vi "test Get Attribute as DBL2.vi"(11 "Test Case In":refnum<class "Test Config From Excel Table.lvclass">) -> (0 "error out":errorcluster, 3 "Test Case Out":refnum<class "Test Config From Excel Table.lvclass">)   [LabVIEW 2020, in "Test Config From Excel Table.lvclass"]
uses:
  Test Config From Excel Table.lvclass
  C:/Program Files/National Instruments/LabVIEW 2025/vi.lib/Astemes/LUnit/Test Case.lvclass
  Source/Config from Excel Table/Config from Excel Table.lvclass
  <vilib>/Astemes/LUnit/Test Case.lvclass/Test Case.ctl
  <vilib>/Astemes/LUnit/Test Case.lvclass
  Open-Xml-LabVIEW/Source/Open Xml.lvlib
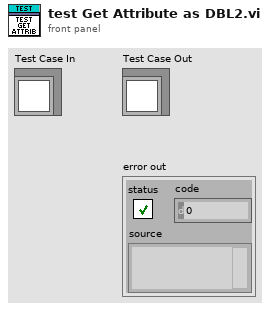
[diagram p1: front panel]
types:
  T1 = cluster{"Sheet Name":string, "Name":string, "Display Name":string, "Range or Cell Address":string}
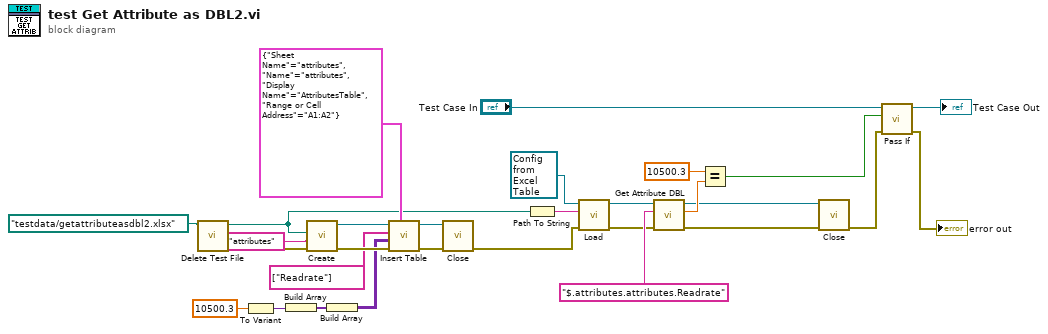
[diagram p0: block diagram]
diagram:
  n1 = call "Delete Test File.vi"("name or relative path"=path "testdata/getattributeasdbl2.xlsx") -> ("error out"=w15:errorcluster, "deleted path"=w3:path)  [unwired: 9 in]
  n2 = To Variant(anything=10500.3) -> (Variant=w9:variant)
  n3 = Build Array(w9) -> (w8:variant[])
  n4 = call "Create.vi"("error in"=w15, "SheetName"="attributes", "Path"=w3) -> ("error out"=w14:errorcluster, "SpreadsheetDoc"=w6:refnum<k24>)  [unwired: 7 in]
  n5 = Build Array(w8) -> (w7:variant[][])
  n6 = call "Insert Table.vi"("Location"=T1 {"Sheet Name"="attributes", "Name"="attributes", "Display Name"="AttributesTable", "Range or Cell Address"="A1:A2"}, "error in"=w14, "Cell Values"=w7, "Header Names"=string[] ["Readrate"], "SpreadsheetDoc in"=w6) -> ("error out"=w13:errorcluster, "SpreadsheetDoc out"=w4:refnum<k24>)  [unwired: 5 in]
  n7 = call "Close.vi"("error in"=w13, "SpreadsheetDoc"=w4) -> ("error out"=w5:errorcluster)  [unwired: 9 in]
  n8 = Path To String(path=w3) -> (string=w25:string)
  n9 = call-dynamic "Load.vi"("error in"=w5, "Source"=w25, "Config from Excel Table in"=refnum<class "Config from Excel Table.lvclass"> refnum ("Config from EXCEL Table.lvclass")) -> ("error out"=w16:errorcluster, "Config from Excel Table out"=w17:refnum<class "Config from Excel Table.lvclass">)  [unwired: 7 in]
  n10 = call-dynamic "Get Attribute DBL.vi"("error in"=w16, "Attribute"="$.attributes.attributes.Readrate", "Config from Excel Table in"=w17) -> ("error out"=w19:errorcluster, "Value"=w22:dbl, "Config from Excel Table out"=w20:refnum<class "Config from Excel Table.lvclass">)  [unwired: 6 in]
  n11 = Equal?(x=10500.3 ("Value"), y=w22) -> (x = y?=w21:bool)
  n12 = call-dynamic "Close.vi"("error in"=w19, "Config from Excel Table in"=w20) -> ("error out"=w18:errorcluster)  [unwired: 8 in, 1 out]
  n13 = call <vilib>:"Pass If.vi"("error in (no error)"=w18, "Pass?"=w21, "LUnit Test Case In"="Test Case In") -> ("error out"=→"error out":errorcluster, "LUnit Test Case Out"=→"Test Case Out":refnum<class "Test Config From Excel Table.lvclass">)  [unwired: 7 in]
